vi "WildDrive_v5.vi"(6 "Selected_Driver":i32=3, 8 "Super Turn":bool, 9 "Legal_Drivers":string[](array[string])=["Ethan", "Adam", "Amelia", "Safety Drive"], 10 "Turn Joystick":dbl, 11 "Speed Joystick":dbl=-0.0) -> (0 "Right Side Power":dbl, 3 "Left Side Power":dbl)   [LabVIEW 2018]
uses:
  <vilib>/Analysis/1siggen.llb/Ramp Pattern by Samples.vi
  <vilib>/Analysis/NI_AALBase.lvlib
panel:
  in  "Max Speed":dbl[](array[slide])=[1.0, 1.0, 1.0, 0.25] min=0.0 max=1.0 scale=0.0..1.0
  in  "Sync Driver Profile":bool
  out "Current_Driver":string="Safety Drive"
  in  "Feed Forward Coeff":dbl[](array[slide])=[0.05, 0.05, 0.05, 0.019999999999999997] min=0.0 max=0.2 scale=0.0..0.2
  in  "Mixing Coefficient":dbl[](array[slide])=[20.0, 20.0, 25.0, 20.0] min=1.0 max=100.0 scale=1.0..100.0
  in  "Max Pivot Turn (super)":dbl[](array[slide])=[1.0, 1.0, 1.0, 0.0] min=0.0 max=1.0 scale=0.0..1.0
  in  "Max Pivot Turn (normal)":dbl[](array[slide])=[0.8, 0.8, 0.5, 0.8] min=0.0 max=1.0 scale=0.0..1.0
  in  "Tune Arc Turn":dbl[](array[slide])=[1.2, 1.2, 0.9, 1.2] min=0.9 max=2.0 scale=0.9..2.0
  in  "Speed Joystick Deadband":dbl[](array[slide])=[0.05, 0.05, 0.05, 0.6] min=0.0 max=1.0 scale=0.0..1.0
  in  "Turning Joystick Deadband":dbl[](array[slide])=[0.05, 0.1, 0.2, 0.3] min=0.0 max=1.0 scale=0.0..1.0
  out "Mixing Function":cluster{"Y":dbl[], "X":dbl[]}(graph)={"Y"=[0.0, 0.010101010101010102, 0.020202020202020204, 0.030303030303030304, 0.04040404040404041, 0.05050505050505051, 0.06060606060606061, 0.07070707070707072, 0.08080808080808081, 0.09090909090909091, 0.10101010101010102, 0.11111111111111112, 0.12121212121212122, 0.13131313131313133, 0.14141414141414144, 0.15151515151515152, 0.16161616161616163, 0.17171717171717174, 0.18181818181818182, 0.19191919191919193, 0.20202020202020204, 0.21212121212121213, 0.22222222222222224, 0.23232323232323235, 0.24242424242424243, 0.25252525252525254, 0.26262626262626265, 0.27272727272727276, 0.2828282828282829, 0.29292929292929293, 0.30303030303030304, 0.31313131313131315, 0.32323232323232326, 0.33333333333333337, 0.3434343434343435, 0.3535353535353536, 0.36363636363636365, 0.37373737373737376, 0.38383838383838387, 0.393939393939394, 0.4040404040404041, 0.4141414141414142, 0.42424242424242425, 0.43434343434343436, 0.4444444444444445, 0.4545454545454546, 0.4646464646464647, 0.4747474747474748, 0.48484848484848486, 0.494949494949495, 0.5050505050505051, 0.5151515151515152, 0.5252525252525253, 0.5353535353535354, 0.5454545454545455, 0.5555555555555556, 0.5656565656565657, 0.5757575757575758, 0.5858585858585859, 0.595959595959596, 0.6060606060606061, 0.6161616161616162, 0.6262626262626263, 0.6363636363636365, 0.6464646464646465, 0.6565656565656566, 0.6666666666666667, 0.6767676767676768, 0.686868686868687, 0.696969696969697, 0.7070707070707072, 0.7171717171717172, 0.7272727272727273, 0.7373737373737375, 0.7474747474747475, 0.7575757575757577, 0.7676767676767677, 0.7777777777777778, 0.787878787878788, 0.797979797979798, 0.8080808080808082, 0.8181818181818182, 0.8282828282828284, 0.8383838383838385, 0.8484848484848485, 0.8585858585858587, 0.8686868686868687, 0.8787878787878789, 0.888888888888889, 0.8989898989898991, 0.9090909090909092, 0.9191919191919192, 0.9292929292929294, 0.9393939393939394, 0.9494949494949496, 0.9595959595959597, 0.9696969696969697, 0.9797979797979799, 0.98989898989899, 1.0], "X"=[1.0, 0.36603234127322715, 0.13532626064379283, 0.05052453015628186, 0.019045702193466962, 0.007247455040202033, 0.002783489278110511, 0.0010787801167675484, 0.00042183410694076207, 0.00016639639425326962, 6.620177984839095e-05, 2.6561398887587357e-05, 1.0745375115522577e-05, 4.382452248980866e-06, 1.8016694372108035e-06, 7.465077591438598e-07, 3.1169901107319554e-07, 1.3113557868070773e-07, 5.5581886768235786e-08, 2.373114697909272e-08, 1.0205242300096137e-08, 4.419721001217318e-09, 1.927446925622597e-09, 8.463234846310681e-10, 3.7411775176233565e-10, 1.6647573596881723e-10, 7.456210476755159e-11, 3.360972414714873e-11, 1.5245699808641053e-11, 6.958609969858144e-12, 3.195570695186819e-12, 1.4763326653758367e-12, 6.86103909791559e-13, 3.2072021853814684e-13, 1.5078403574264123e-13, 7.129180709244532e-14, 3.3895544142624165e-14, 1.6204238353260086e-14, 7.788659967873636e-15, 3.76366378038304e-15, 1.82826621688999e-15, 8.927212895741967e-16, 4.381352486286385e-16, 2.1611505485274178e-16, 1.0713113677174099e-16, 5.336668792886832e-17, 2.6712789155004126e-17, 1.3434882772756658e-17, 6.788690117455716e-18, 3.4462590553247523e-18, 1.7574890123257356e-18, 9.003130684840785e-19, 4.632599227711995e-19, 2.394201316530436e-19, 1.2427288424976475e-19, 6.478095947844572e-20, 3.391170633552417e-20, 1.782623487107148e-20, 9.409232908362009e-21, 4.986671552400837e-21, 2.6534262895136237e-21, 1.4174938853880581e-21, 7.602069865092925e-22, 4.0927762769197154e-22, 2.211867051717034e-22, 1.1998712710421777e-22, 6.53318623500068e-23, 3.570348880574086e-23, 1.958268982155976e-23, 1.0779318073480446e-23, 5.95455071339927e-24, 3.300861649468989e-24, 1.8361511142543956e-24, 1.0248841317144169e-24, 5.739963712987115e-25, 3.2254820658410615e-25, 1.8185053837023498e-25, 1.0286145857915951e-25, 5.837042071494194e-26, 3.3229149745670054e-26, 1.8976510791597504e-26, 1.0870986324891945e-26, 6.246862874883761e-27, 3.6006479544686514e-27, 2.0816633052912476e-27, 1.2070830701485794e-27, 7.020153679465042e-28, 4.094727808938361e-28, 2.3952938868546393e-28, 1.4051883268944269e-28, 8.266830677466088e-29, 4.877074216359946e-29, 2.8852452517622416e-29, 1.711577581520392e-29, 1.0180955963877349e-29, 6.0722055822989395e-30, 3.6312681754960745e-30, 2.1772701780581707e-30, 1.3088709946601708e-30, 7.888609052210118e-31]}
  in  "Debug Mode":bool
  in  "Debug Speed":dbl(slide) min=0.0 max=1.0 scale=0.0..1.0
  in  "Square Speed":bool=TRUE
  in  "Turn Behavior":bool=TRUE
  out "Left Side Power":cluster{"Y":dbl[], "X":dbl[]}(graph)={"Y"=[0.0, 0.010101010101010102, 0.020202020202020204, 0.030303030303030304, 0.04040404040404041, 0.05050505050505051, 0.06060606060606061, 0.07070707070707072, 0.08080808080808081, 0.09090909090909091, 0.10101010101010102, 0.11111111111111112, 0.12121212121212122, 0.13131313131313133, 0.14141414141414144, 0.15151515151515152, 0.16161616161616163, 0.17171717171717174, 0.18181818181818182, 0.19191919191919193, 0.20202020202020204, 0.21212121212121213, 0.22222222222222224, 0.23232323232323235, 0.24242424242424243, 0.25252525252525254, 0.26262626262626265, 0.27272727272727276, 0.2828282828282829, 0.29292929292929293, 0.30303030303030304, 0.31313131313131315, 0.32323232323232326, 0.33333333333333337, 0.3434343434343435, 0.3535353535353536, 0.36363636363636365, 0.37373737373737376, 0.38383838383838387, 0.393939393939394, 0.4040404040404041, 0.4141414141414142, 0.42424242424242425, 0.43434343434343436, 0.4444444444444445, 0.4545454545454546, 0.4646464646464647, 0.4747474747474748, 0.48484848484848486, 0.494949494949495, 0.5050505050505051, 0.5151515151515152, 0.5252525252525253, 0.5353535353535354, 0.5454545454545455, 0.5555555555555556, 0.5656565656565657, 0.5757575757575758, 0.5858585858585859, 0.595959595959596, 0.6060606060606061, 0.6161616161616162, 0.6262626262626263, 0.6363636363636365, 0.6464646464646465, 0.6565656565656566, 0.6666666666666667, 0.6767676767676768, 0.686868686868687, 0.696969696969697, 0.7070707070707072, 0.7171717171717172, 0.7272727272727273, 0.7373737373737375, 0.7474747474747475, 0.7575757575757577, 0.7676767676767677, 0.7777777777777778, 0.787878787878788, 0.797979797979798, 0.8080808080808082, 0.8181818181818182, 0.8282828282828284, 0.8383838383838385, 0.8484848484848485, 0.8585858585858587, 0.8686868686868687, 0.8787878787878789, 0.888888888888889, 0.8989898989898991, 0.9090909090909092, 0.9191919191919192, 0.9292929292929294, 0.9393939393939394, 0.9494949494949496, 0.9595959595959597, 0.9696969696969697, 0.9797979797979799, 0.98989898989899, 1.0], "X"=[0.0]}
  out "Right Side Power":cluster{"Y":dbl[], "X":dbl[]}(graph)={"Y"=[0.0, 0.010101010101010102, 0.020202020202020204, 0.030303030303030304, 0.04040404040404041, 0.05050505050505051, 0.06060606060606061, 0.07070707070707072, 0.08080808080808081, 0.09090909090909091, 0.10101010101010102, 0.11111111111111112, 0.12121212121212122, 0.13131313131313133, 0.14141414141414144, 0.15151515151515152, 0.16161616161616163, 0.17171717171717174, 0.18181818181818182, 0.19191919191919193, 0.20202020202020204, 0.21212121212121213, 0.22222222222222224, 0.23232323232323235, 0.24242424242424243, 0.25252525252525254, 0.26262626262626265, 0.27272727272727276, 0.2828282828282829, 0.29292929292929293, 0.30303030303030304, 0.31313131313131315, 0.32323232323232326, 0.33333333333333337, 0.3434343434343435, 0.3535353535353536, 0.36363636363636365, 0.37373737373737376, 0.38383838383838387, 0.393939393939394, 0.4040404040404041, 0.4141414141414142, 0.42424242424242425, 0.43434343434343436, 0.4444444444444445, 0.4545454545454546, 0.4646464646464647, 0.4747474747474748, 0.48484848484848486, 0.494949494949495, 0.5050505050505051, 0.5151515151515152, 0.5252525252525253, 0.5353535353535354, 0.5454545454545455, 0.5555555555555556, 0.5656565656565657, 0.5757575757575758, 0.5858585858585859, 0.595959595959596, 0.6060606060606061, 0.6161616161616162, 0.6262626262626263, 0.6363636363636365, 0.6464646464646465, 0.6565656565656566, 0.6666666666666667, 0.6767676767676768, 0.686868686868687, 0.696969696969697, 0.7070707070707072, 0.7171717171717172, 0.7272727272727273, 0.7373737373737375, 0.7474747474747475, 0.7575757575757577, 0.7676767676767677, 0.7777777777777778, 0.787878787878788, 0.797979797979798, 0.8080808080808082, 0.8181818181818182, 0.8282828282828284, 0.8383838383838385, 0.8484848484848485, 0.8585858585858587, 0.8686868686868687, 0.8787878787878789, 0.888888888888889, 0.8989898989898991, 0.9090909090909092, 0.9191919191919192, 0.9292929292929294, 0.9393939393939394, 0.9494949494949496, 0.9595959595959597, 0.9696969696969697, 0.9797979797979799, 0.98989898989899, 1.0], "X"=[0.0]}
  out "Speed Joystick Mapping":cluster{"Y":dbl[], "X":dbl[]}(graph)={"Y"=[0.0, 0.010101010101010102, 0.020202020202020204, 0.030303030303030304, 0.04040404040404041, 0.05050505050505051, 0.06060606060606061, 0.07070707070707072, 0.08080808080808081, 0.09090909090909091, 0.10101010101010102, 0.11111111111111112, 0.12121212121212122, 0.13131313131313133, 0.14141414141414144, 0.15151515151515152, 0.16161616161616163, 0.17171717171717174, 0.18181818181818182, 0.19191919191919193, 0.20202020202020204, 0.21212121212121213, 0.22222222222222224, 0.23232323232323235, 0.24242424242424243, 0.25252525252525254, 0.26262626262626265, 0.27272727272727276, 0.2828282828282829, 0.29292929292929293, 0.30303030303030304, 0.31313131313131315, 0.32323232323232326, 0.33333333333333337, 0.3434343434343435, 0.3535353535353536, 0.36363636363636365, 0.37373737373737376, 0.38383838383838387, 0.393939393939394, 0.4040404040404041, 0.4141414141414142, 0.42424242424242425, 0.43434343434343436, 0.4444444444444445, 0.4545454545454546, 0.4646464646464647, 0.4747474747474748, 0.48484848484848486, 0.494949494949495, 0.5050505050505051, 0.5151515151515152, 0.5252525252525253, 0.5353535353535354, 0.5454545454545455, 0.5555555555555556, 0.5656565656565657, 0.5757575757575758, 0.5858585858585859, 0.595959595959596, 0.6060606060606061, 0.6161616161616162, 0.6262626262626263, 0.6363636363636365, 0.6464646464646465, 0.6565656565656566, 0.6666666666666667, 0.6767676767676768, 0.686868686868687, 0.696969696969697, 0.7070707070707072, 0.7171717171717172, 0.7272727272727273, 0.7373737373737375, 0.7474747474747475, 0.7575757575757577, 0.7676767676767677, 0.7777777777777778, 0.787878787878788, 0.797979797979798, 0.8080808080808082, 0.8181818181818182, 0.8282828282828284, 0.8383838383838385, 0.8484848484848485, 0.8585858585858587, 0.8686868686868687, 0.8787878787878789, 0.888888888888889, 0.8989898989898991, 0.9090909090909092, 0.9191919191919192, 0.9292929292929294, 0.9393939393939394, 0.9494949494949496, 0.9595959595959597, 0.9696969696969697, 0.9797979797979799, 0.98989898989899, 1.0], "X"=[0.0]}
  out "Turn Joystick Mapping":cluster{"Y":dbl[], "X":dbl[]}(graph)={"Y"=[0.0, 0.010101010101010102, 0.020202020202020204, 0.030303030303030304, 0.04040404040404041, 0.05050505050505051, 0.06060606060606061, 0.07070707070707072, 0.08080808080808081, 0.09090909090909091, 0.10101010101010102, 0.11111111111111112, 0.12121212121212122, 0.13131313131313133, 0.14141414141414144, 0.15151515151515152, 0.16161616161616163, 0.17171717171717174, 0.18181818181818182, 0.19191919191919193, 0.20202020202020204, 0.21212121212121213, 0.22222222222222224, 0.23232323232323235, 0.24242424242424243, 0.25252525252525254, 0.26262626262626265, 0.27272727272727276, 0.2828282828282829, 0.29292929292929293, 0.30303030303030304, 0.31313131313131315, 0.32323232323232326, 0.33333333333333337, 0.3434343434343435, 0.3535353535353536, 0.36363636363636365, 0.37373737373737376, 0.38383838383838387, 0.393939393939394, 0.4040404040404041, 0.4141414141414142, 0.42424242424242425, 0.43434343434343436, 0.4444444444444445, 0.4545454545454546, 0.4646464646464647, 0.4747474747474748, 0.48484848484848486, 0.494949494949495, 0.5050505050505051, 0.5151515151515152, 0.5252525252525253, 0.5353535353535354, 0.5454545454545455, 0.5555555555555556, 0.5656565656565657, 0.5757575757575758, 0.5858585858585859, 0.595959595959596, 0.6060606060606061, 0.6161616161616162, 0.6262626262626263, 0.6363636363636365, 0.6464646464646465, 0.6565656565656566, 0.6666666666666667, 0.6767676767676768, 0.686868686868687, 0.696969696969697, 0.7070707070707072, 0.7171717171717172, 0.7272727272727273, 0.7373737373737375, 0.7474747474747475, 0.7575757575757577, 0.7676767676767677, 0.7777777777777778, 0.787878787878788, 0.797979797979798, 0.8080808080808082, 0.8181818181818182, 0.8282828282828284, 0.8383838383838385, 0.8484848484848485, 0.8585858585858587, 0.8686868686868687, 0.8787878787878789, 0.888888888888889, 0.8989898989898991, 0.9090909090909092, 0.9191919191919192, 0.9292929292929294, 0.9393939393939394, 0.9494949494949496, 0.9595959595959597, 0.9696969696969697, 0.9797979797979799, 0.98989898989899, 1.0], "X"=[-0.0]}
  # "Driver Inputs"
  # "Tuning Parameters"
  # "Debug"
  # "Drive Outputs"
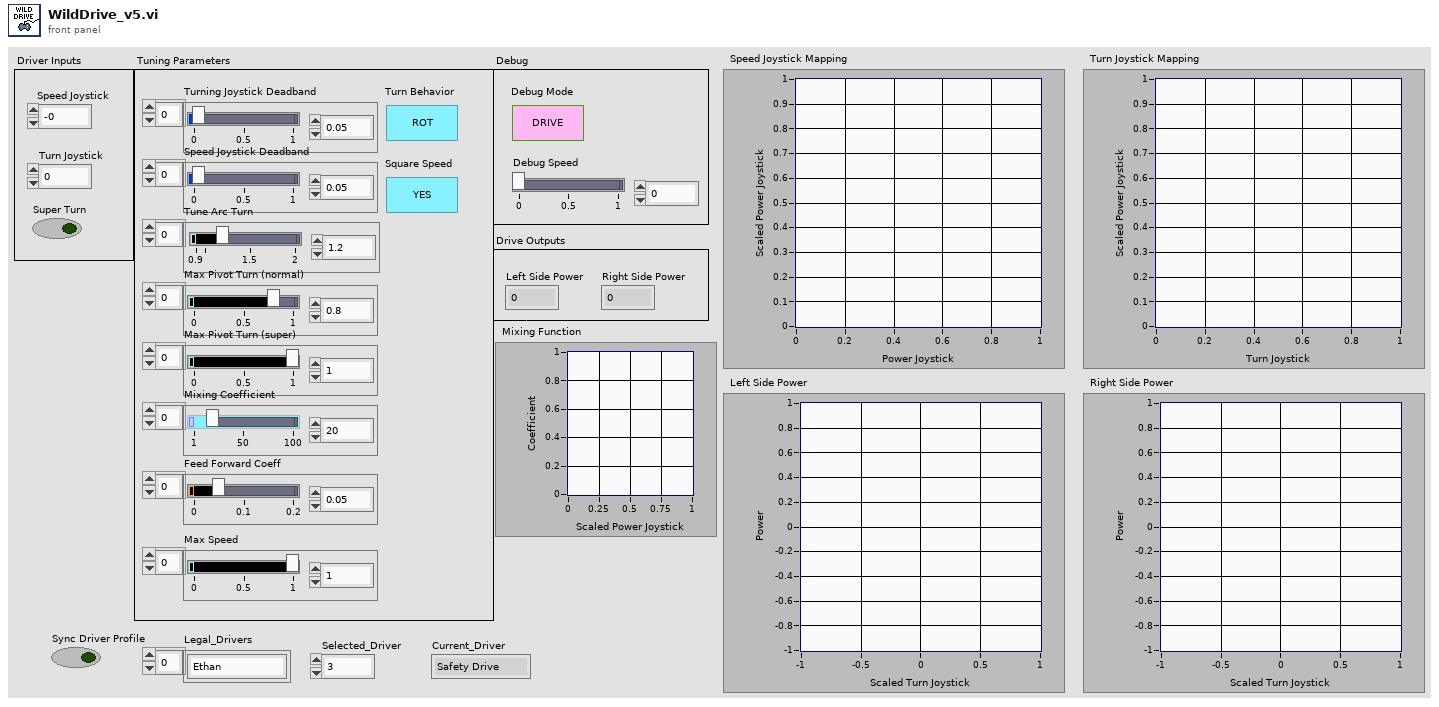
[diagram p1: front panel]
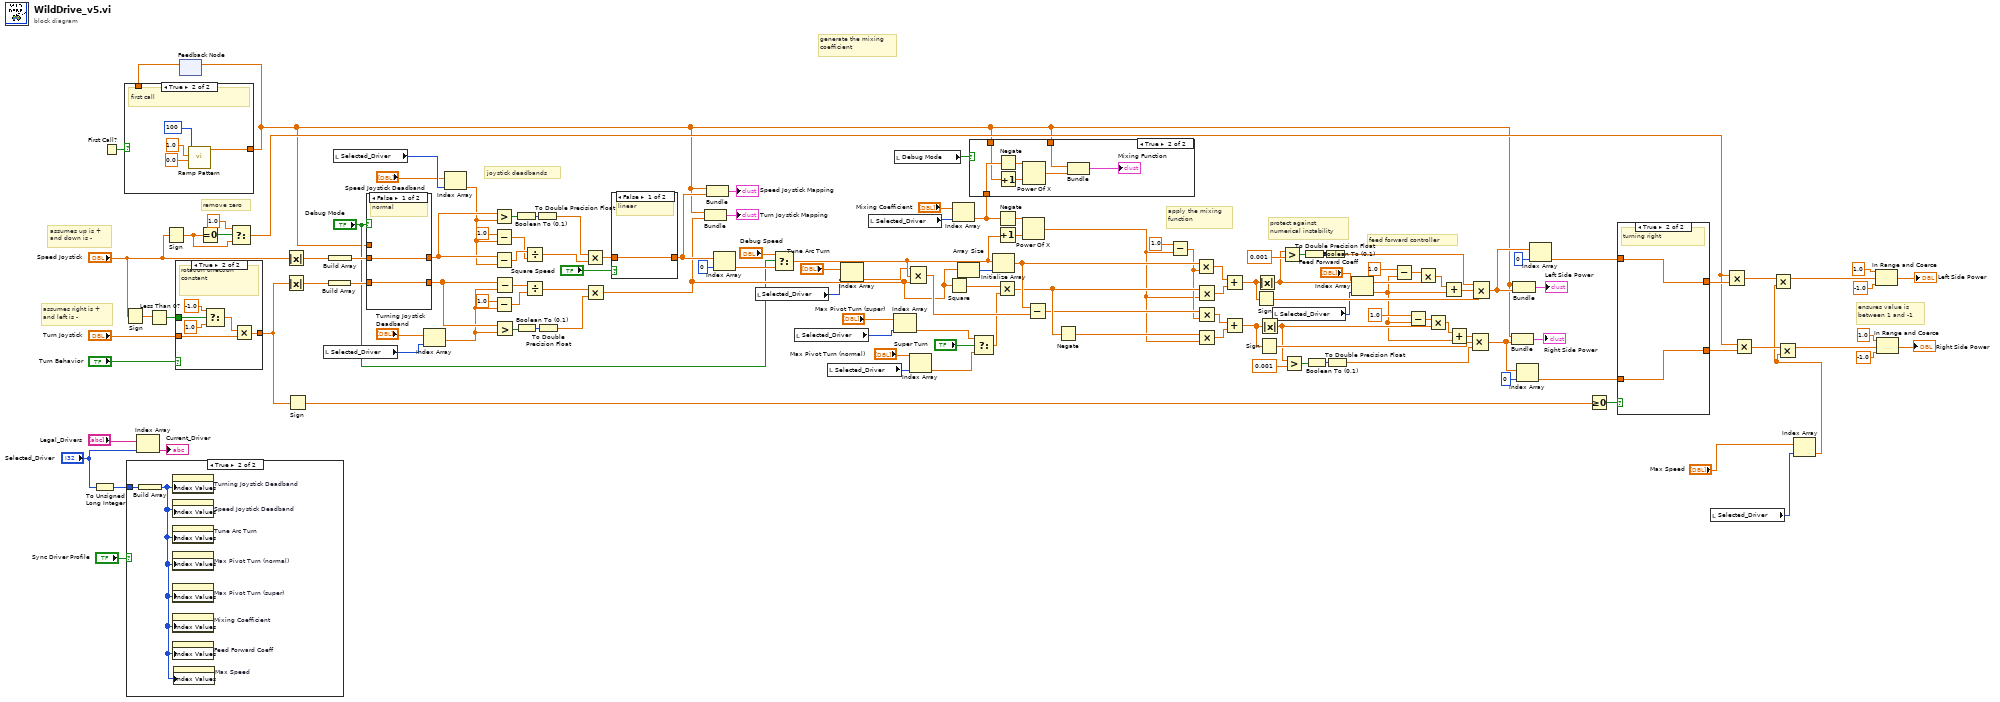
[diagram p0: block diagram]
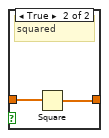
[diagram p8: hidden frame]
diagram:
  # "assumes right is +\nand left is -"
  # "assumes up is +\nand down is -"
  # "apply the mixing\nfunction"
  # "generate the mixing\ncoefficient"
  # "remove zero"
  # "protect against\nnumerical instability"
  # "ensures value is \nbetween 1 and -1"
  # "feed forward controller"
  # "joystick deadbands"
  n1 = To Unsigned Long Integer(number="Selected_Driver") -> (unsigned 32bit integer=w7:u32)
  n2 = First Call?() -> (First Call?: T/F=w57:bool)
  n3 = Sign(1:"Speed Joystick") -> (0:w67:dbl)
  n4 = case shown="True" "Sync Driver Profile" {
    tunnel: w7 -> [_ w138]
    frame False {
    }
    frame True {
      n5 = Build Array(w138) -> (w137:u32[])
      n6 = property on="Turning Joystick Deadband" class="Arr (strict)"("Index Values"=w137) -> ()  [unwired: 2 in, 2 out]
      n7 = property on="Speed Joystick Deadband" class="Arr (strict)"("Index Values"=w137) -> ()  [unwired: 2 in, 2 out]
      n8 = property on="Tune Arc Turn" class="Arr (strict)"("Index Values"=w137) -> ()  [unwired: 2 in, 2 out]
      n9 = property on="Max Pivot Turn (normal)" class="Arr (strict)"("Index Values"=w137) -> ()  [unwired: 2 in, 2 out]
      n10 = property on="Max Pivot Turn (super)" class="Arr (strict)"("Index Values"=w137) -> ()  [unwired: 2 in, 2 out]
      n11 = property on="Mixing Coefficient" class="Arr (strict)"("Index Values"=w137) -> ()  [unwired: 2 in, 2 out]
      n12 = property on="Feed Forward Coeff" class="Arr (strict)"("Index Values"=w137) -> ()  [unwired: 2 in, 2 out]
      n13 = property on="Max Speed" class="Arr (strict)"("Index Values"=w137) -> ()  [unwired: 2 in, 2 out]
    }
  }
  n14 = Index Array(array="Legal_Drivers", index="Selected_Driver") -> (element=→"Current_Driver":string)
  n15 = Less Than 0?(x=w67) -> (x < 0?=w68:bool)
  n16 = Sign(1:"Speed Joystick") -> (0:w60:dbl)
  n17 = case shown="True" "Turn Behavior" {
    tunnel: w68 -> [_ w144]
    tunnel: [w139 w141] -> w63
    tunnel: "Turn Joystick" -> [w139 w140]
    frame False {
      # "like a car"
    }
    frame True {
      # "rotation direction constant"
      n18 = Select(t=-1.0, s=w144, f=1.0) -> (s? t:f=w145:dbl)
      n19 = Multiply(x=w145, y=w140) -> (x*y=w141:dbl)
    }
  }
  n20 = feedback #1() -> (w56:dbl[])  [unwired: 1 in]
  n21 = case shown="True" w57 {
    tunnel: [w146 w147] -> w33
    tunnel: w56 -> [w146 _]
    frame False {
      # "subsequent calls"
    }
    frame True {
      # "first call"
      n22 = call-poly <vilib>:"Ramp Pattern.vi"("start"=0.0, "end"=1.0, "samples"=100) -> ("Ramp Pattern"=w147:dbl[])  [unwired: 7 in, 1 out]
    }
  }
  n23 = feedback-in #1(w33) -> ()
  n24 = Equal To 0?(x=w60) -> (x = 0?=w62:bool)
  n25 = Select(t=1.0, s=w62, f=w60) -> (s? t:f=w59:dbl)
  n26 = Absolute Value(x="Speed Joystick") -> (abs(x)=w133:dbl)
  n27 = Absolute Value(x=w63) -> (abs(x)=w136:dbl)
  n28 = Sign(1:w63) -> (0:w71:dbl)
  n29 = local read "Selected_Driver"() -> (w29:i32)
  n30 = Build Array(w136) -> (w134:dbl[])
  n31 = Build Array(w133) -> (w135:dbl[])
  n32 = local read "Selected_Driver"() -> (w28:i32)
  n33 = case shown="False" "Debug Mode" {
    tunnel: w33 -> [_ w153]
    tunnel: [w152 w153] -> w124
    tunnel: [w151 w153] -> w116
    tunnel: w135 -> [w152 _]
    tunnel: w134 -> [w151 _]
    frame False {
      # "normal"
    }
    frame True {
      # "debug"
    }
  }
  n34 = Index Array(array="Turning Joystick Deadband", index=w29) -> (element=w30:dbl)
  n35 = Index Array(array="Speed Joystick Deadband", index=w28) -> (element=w27:dbl)
  n36 = Greater?(x=w124, y=w27) -> (0:w130:bool[])
  n37 = Subtract(x=1.0, y=w27) -> (x-y=w121:dbl)
  n38 = Subtract(x=w124, y=w27) -> (x-y=w123:dbl[])
  n39 = Subtract(x=1.0, y=w30) -> (x-y=w117:dbl)
  n40 = Subtract(x=w116, y=w30) -> (x-y=w119:dbl[])
  n41 = Greater?(x=w116, y=w30) -> (0:w128:bool[])
  n42 = Boolean To (0,1)(Boolean=w130) -> (0, 1=w129:i16[])
  n43 = Boolean To (0,1)(Boolean=w128) -> (0, 1=w127:i16[])
  n44 = Divide(x=w123, y=w121) -> (x/y=w120:dbl[])
  n45 = Divide(x=w119, y=w117) -> (x/y=w115:dbl[])
  n46 = To Double Precision Float(number=w129) -> (double precision float=w126:dbl[])
  n47 = To Double Precision Float(number=w127) -> (double precision float=w114:dbl[])
  n48 = Multiply(x=w126, y=w120) -> (x*y=w125:dbl[])
  n49 = Multiply(x=w115, y=w114) -> (x*y=w52:dbl[])
  n50 = case shown="False" "Square Speed" {
    tunnel: w125 -> [w154 w156]
    tunnel: [w154 w155] -> w107
    frame False {
      # "linear"
    }
    frame True {
      # "squared"
      n51 = Square(x=w156) -> (x^2=w155:dbl[])
    }
  }
  n52 = Bundle("Ramp Pattern"=w33, w52) -> (→"Turn Joystick Mapping":cluster{"Ramp Pattern":dbl[], dbl[]})  [unwired: 1 in]
  n53 = Bundle("Ramp Pattern"=w33, w107) -> (→"Speed Joystick Mapping":cluster{"Ramp Pattern":dbl[], dbl[]})  [unwired: 1 in]
  n54 = Index Array(array=w107, index=0) -> (element=w109:dbl)
  n55 = local read "Selected_Driver"() -> (w24:i32)
  n56 = Select(t="Debug Speed", s="Debug Mode", f=w109) -> (s? t:f=w37:dbl)
  n57 = local read "Selected_Driver"() -> (w18:i32)
  n58 = local read "Selected_Driver"() -> (w22:i32)
  n59 = Index Array(array="Tune Arc Turn", index=w24) -> (element=w23:dbl)
  n60 = local read "Selected_Driver"() -> (w14:i32)
  n61 = Index Array(array="Max Pivot Turn (super)", index=w18) -> (element=w17:dbl)
  n62 = local read "Debug Mode"() -> (w32:bool)
  n63 = Index Array(array="Max Pivot Turn (normal)", index=w22) -> (element=w20:dbl)
  n64 = Compound Arithmetic op=MULTIPLY(w23, w37, w52) -> (w110:dbl[])
  n65 = Square(x=w52) -> (x^2=w58:dbl[])
  n66 = Index Array(array="Mixing Coefficient", index=w14) -> (element=w16:dbl)
  n67 = Array Size(array=w52) -> (size(s)=w113:i32)
  n68 = case shown="True" w32 {
    tunnel: w16 -> [_ w161]
    tunnel: w33 -> [_ w159]
    tunnel: w33 -> [_ w157]
    frame False {
    }
    frame True {
      n69 = Negate(x=w161) -> (-x=w163:dbl)
      n70 = Increment(x=w159) -> (x+1=w162:dbl[])
      n71 = Power Of X(1:w162, 2:w163) -> (0:w158:dbl[])
      n72 = Bundle("Ramp Pattern"=w157, w158) -> (→"Mixing Function":cluster{"Ramp Pattern":dbl[], dbl[]})  [unwired: 1 in]
    }
  }
  n73 = Select(t=w17, s="Super Turn", f=w20) -> (s? t:f=w55:dbl)
  n74 = Initialize Array(w37, w113) -> (w49:dbl[])
  n75 = Multiply(x=w58, y=w55) -> (x*y=w48:dbl[])
  n76 = Negate(x=w16) -> (-x=w36:dbl)
  n77 = Increment(x=w37) -> (x+1=w35:dbl)
  n78 = Power Of X(1:w35, 2:w36) -> (0:w34:dbl)
  n79 = Subtract(x=w49, y=w110) -> (x-y=w42:dbl[])
  n80 = Negate(x=w48) -> (-x=w41:dbl[])
  n81 = Subtract(x=1.0, y=w34) -> (x-y=w38:dbl)
  n82 = Multiply(x=w49, y=w38) -> (x*y=w47:dbl[])
  n83 = Multiply(x=w48, y=w34) -> (x*y=w46:dbl[])
  n84 = Multiply(x=w42, y=w38) -> (x*y=w44:dbl[])
  n85 = Multiply(x=w41, y=w34) -> (x*y=w43:dbl[])
  n86 = Add(x=w47, y=w46) -> (x+y=w45:dbl[])
  n87 = Add(x=w44, y=w43) -> (x+y=w40:dbl[])
  n88 = Sign(1:w45) -> (0:w103:dbl[])
  n89 = Absolute Value(x=w45) -> (abs(x)=w69:dbl[])
  n90 = Sign(1:w40) -> (0:w98:dbl[])
  n91 = Absolute Value(x=w40) -> (abs(x)=w70:dbl[])
  n92 = local read "Selected_Driver"() -> (w11:i32)
  n93 = Greater?(x=w69, y=0.001) -> (0:w93:bool[])
  n94 = Greater?(x=w70, y=0.001) -> (0:w97:bool[])
  n95 = Boolean To (0,1)(Boolean=w93) -> (0, 1=w92:i16[])
  n96 = Boolean To (0,1)(Boolean=w97) -> (0, 1=w96:i16[])
  n97 = To Double Precision Float(number=w92) -> (double precision float=w90:dbl[])
  n98 = To Double Precision Float(number=w96) -> (double precision float=w94:dbl[])
  n99 = Index Array(array="Feed Forward Coeff", index=w11) -> (element=w13:dbl)
  n100 = Subtract(x=1.0, y=w13) -> (x-y=w105:dbl)
  n101 = Subtract(x=1.0, y=w13) -> (x-y=w101:dbl)
  n102 = Multiply(x=w105, y=w69) -> (x*y=w104:dbl[])
  n103 = Multiply(x=w101, y=w70) -> (x*y=w100:dbl[])
  n104 = Add(x=w104, y=w13) -> (x+y=w89:dbl[])
  n105 = Add(x=w100, y=w13) -> (x+y=w99:dbl[])
  n106 = Compound Arithmetic op=MULTIPLY(w99, w98, w94) -> (w87:dbl[])
  n107 = Compound Arithmetic op=MULTIPLY(w90, w89, w103) -> (w85:dbl[])
  n108 = Bundle("Ramp Pattern"=w33, w87) -> (→"Right Side Power":cluster{"Ramp Pattern":dbl[], dbl[]})  [unwired: 1 in]
  n109 = Bundle("Ramp Pattern"=w33, w85) -> (→"Left Side Power":cluster{"Ramp Pattern":dbl[], dbl[]})  [unwired: 1 in]
  n110 = Index Array(array=w87, index=0) -> (element=w74:dbl)
  n111 = Index Array(array=w85, index=0) -> (element=w76:dbl)
  n112 = Greater Or Equal To 0?(x=w71) -> (x >= 0?=w72:bool)
  n113 = case shown="True" w72 {
    tunnel: w76 -> [w165 w167]
    tunnel: [w164 w167] -> w75
    tunnel: w74 -> [w164 w166]
    tunnel: [w165 w166] -> w73
    frame False {
      # "turning left"
    }
    frame True {
      # "turning right"
    }
  }
  n114 = local read "Selected_Driver"() -> (w3:i32)
  n115 = Multiply(x=w59, y=w75) -> (x*y=w77:dbl)
  n116 = Multiply(x=w59, y=w73) -> (x*y=w78:dbl)
  n117 = Index Array(array="Max Speed", index=w3) -> (element=w1:dbl)
  n118 = Multiply(x=w77, y=w1) -> (x*y=w5:dbl)
  n119 = Multiply(x=w78, y=w1) -> (x*y=w4:dbl)
  n120 = In Range and Coerce(upper limit=1.0, x=w5, lower limit=-1.0) -> (coerced(x)=→"Left Side Power":dbl)  [unwired: 1 out]
  n121 = In Range and Coerce(upper limit=1.0, x=w4, lower limit=-1.0) -> (coerced(x)=→"Right Side Power":dbl)  [unwired: 1 out]
